vi "SmartMessage.vi"(6 "Operation":enum16{"Start", "Message", "Stop", "Disconnect"}(ring)=enum."Message", 8 "error in (no error)":errorcluster, 9 "Timeout (ms)":i32=-1, 10 "Payload":string, 11 "Command":string) -> (0 "error out":errorcluster, 3 "Response":string)   [LabVIEW 2019, in "MicronTemplateAPIs.lvlib" / "MicronTemplateAPIs.lvclass"]
uses:
  MicronTemplateAPIs.lvclass
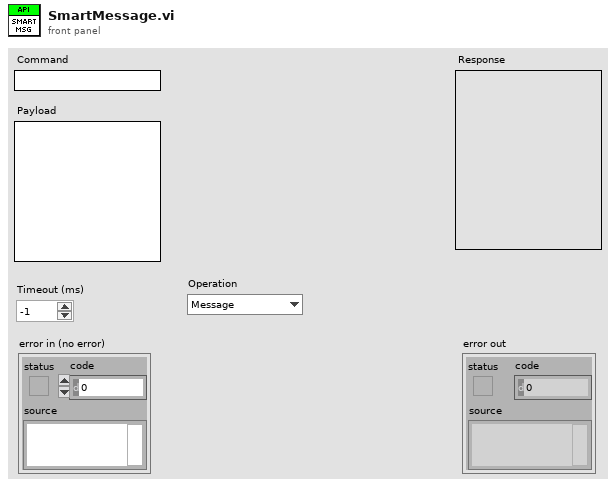
[diagram p1: front panel]
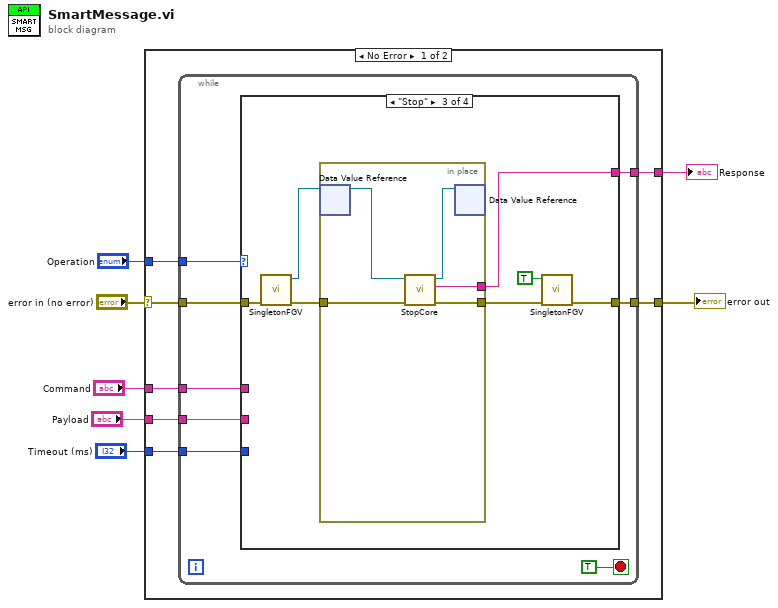
[diagram p0: block diagram]
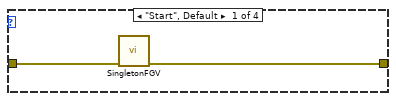
[diagram p2: hidden frame]
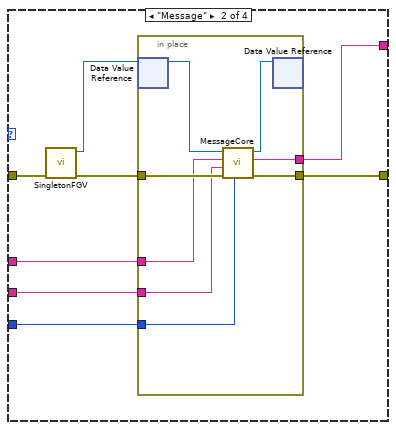
[diagram p3: hidden frame]
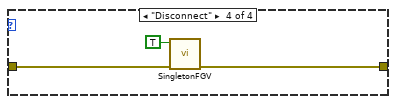
[diagram p4: hidden frame]
diagram:
  n1 = case shown="No Error" "error in (no error)" {
    selector: "error in (no error)" -> [w10 w56]
    tunnel: [w9 w56] -> w6
    tunnel: "Operation" -> [w14 _]
    tunnel: "Command" -> [w13 _]
    tunnel: "Payload" -> [w12 _]
    tunnel: "Timeout (ms)" -> [w11 _]
    tunnel: [w8 _] -> w1
    frame No Error {
      n2 = while {
        tunnel: w14 -> [w21]
        tunnel: w13 -> [w20]
        tunnel: w12 -> [w19]
        tunnel: w11 -> [w18]
        tunnel: w10 -> [w17]
        tunnel: [w16] -> w9
        tunnel: [w15] -> w8
        stop <- TRUE stop-if-true
        n3 = case shown="\"Stop\"" w21 {
          tunnel: w20 -> [_ w28 _ _]
          tunnel: w19 -> [_ w27 _ _]
          tunnel: w18 -> [_ w25 _ _]
          tunnel: w17 -> [w24 w32 w47 w55]
          tunnel: [w23 w30 w42 w53] -> w16
          tunnel: [_ w26 w44 _] -> w15
          frame "Start", Default {
            n4 = call "SingletonFGV.vi"("error in (no error)"=w24) -> ("error out"=w23:errorcluster)  [unwired: 9 in, 1 out]
          }
          frame "Message" {
            n5 = call "SingletonFGV.vi"("error in (no error)"=w32) -> ("error out"=w31:errorcluster, "ServiceClientDVR"=w29:refnum<data-value>)  [unwired: 9 in]
            n6 = in-place {
              in-place-border: w31 -> [w40]
              in-place-border: [w39] -> w30
              in-place-border: w28 -> [w36]
              in-place-border: w27 -> [w35]
              in-place-border: [w34] -> w26
              in-place-border: w25 -> [w33]
              n7 = in-place-dvr #1(w29) -> (w38:refnum<class "MicronTemplateAPIs.lvclass">)  [unwired: 1 out]
              n8 = call-dynamic "MessageCore.vi"("Timeout (ms)"=w33, "error in (no error)"=w40, "Payload"=w35, "Command"=w36, "GRPCClient in"=w38) -> ("error out"=w39:errorcluster, "Response"=w34:string, "GRPCClient out"=w37:refnum<class "MicronTemplateAPIs.lvclass">)  [unwired: 4 in]
              n9 = in-place-dvr #1(w37) -> ()  [unwired: 2 out]
            }
          }
          frame "Stop" {
            n10 = call "SingletonFGV.vi"("error in (no error)"=w47) -> ("error out"=w46:errorcluster, "ServiceClientDVR"=w45:refnum<data-value>)  [unwired: 9 in]
            n11 = in-place {
              in-place-border: w46 -> [w52]
              in-place-border: [w51] -> w43
              in-place-border: [w48] -> w44
              n12 = in-place-dvr #2(w45) -> (w50:refnum<class "MicronTemplateAPIs.lvclass">)  [unwired: 1 out]
              n13 = call-dynamic "StopCore.vi"("error in (no error)"=w52, "MicronClient in"=w50) -> ("error out"=w51:errorcluster, "Response"=w48:string, "MicronClient out"=w49:refnum<class "MicronTemplateAPIs.lvclass">)  [unwired: 7 in]
              n14 = in-place-dvr #2(w49) -> ()  [unwired: 2 out]
            }
            n15 = call "SingletonFGV.vi"("error in (no error)"=w43, "Destroy?"=TRUE) -> ("error out"=w42:errorcluster)  [unwired: 8 in, 1 out]
          }
          frame "Disconnect" {
            n16 = call "SingletonFGV.vi"("error in (no error)"=w55, "Destroy?"=TRUE) -> ("error out"=w53:errorcluster)  [unwired: 8 in, 1 out]
          }
        }
      }
    }
    frame Error {
    }
  }
  "error out" <- w6
  "Response" <- w1
